vi "StartTest.vi"(8 "error in (no error)":errorcluster, 10 "Test":refnum<class "Test.lvclass">, 11 "ResultTreeListener in":refnum<class "ResultTreeListener.lvclass">) -> (0 "error out":errorcluster, 3 "ResultTreeListener out":refnum<class "ResultTreeListener.lvclass">)   [LabVIEW 2017, in "ResultTreeListener.lvclass"]
doc: "A test started."
uses:
  ResultTreeListener.lvclass
  ResultTree/ResultTree.lvclass
  Test/Test.lvclass
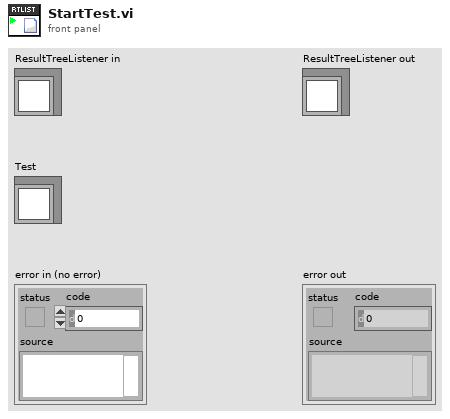
[diagram p1: front panel]
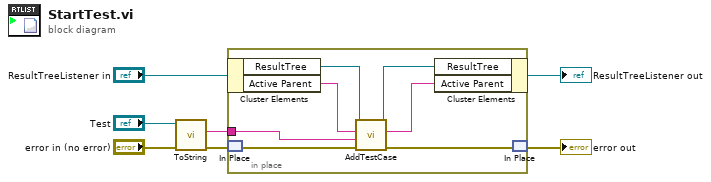
[diagram p0: block diagram]
diagram:
  n1 = call-dynamic "ToString.vi"("error in (no error)"="error in (no error)", "Test In"="Test") -> ("error out"=w6:errorcluster, "String"=w7:string)  [unwired: 7 in, 1 out]
  n2 = in-place {
    in-place-border: w7 -> [w14]
    n3 = in-place-cluster #1("ResultTreeListener in") -> ("ResultTree"=w13:refnum<class "ResultTree.lvclass">, "Active Parent"=w9:string)
    n4 = in-place-match #2(w6) -> (w11:errorcluster)
    n5 = call "AddTestCase.vi"("error in (no error)"=w11, "Name"=w14, "Parent Tag (\"\")"=w9, "ResultTree in"=w13) -> ("error out"=w10:errorcluster, "Tag"=w8:string, "ResultTree out"=w12:refnum<class "ResultTree.lvclass">)  [unwired: 5 in]
    n6 = in-place-cluster #1("ResultTree"=w12, "Active Parent"=w8) -> (→"ResultTreeListener out":refnum<class "ResultTreeListener.lvclass">)
    n7 = in-place-match #2(w10) -> (→"error out":errorcluster)
  }
